vi "SUB-Calculation_Scale_of_CDC_by_data.vi"(10 "MAX r":dbl format="%#.6g", 11 "MIN r":dbl format="%#.6g") -> (3 "Scale(CDC)":dbl format="%#.6g")   [LabVIEW 2015]
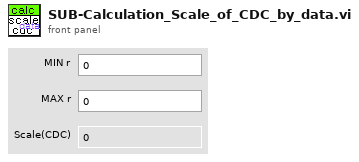
[diagram p1: front panel]
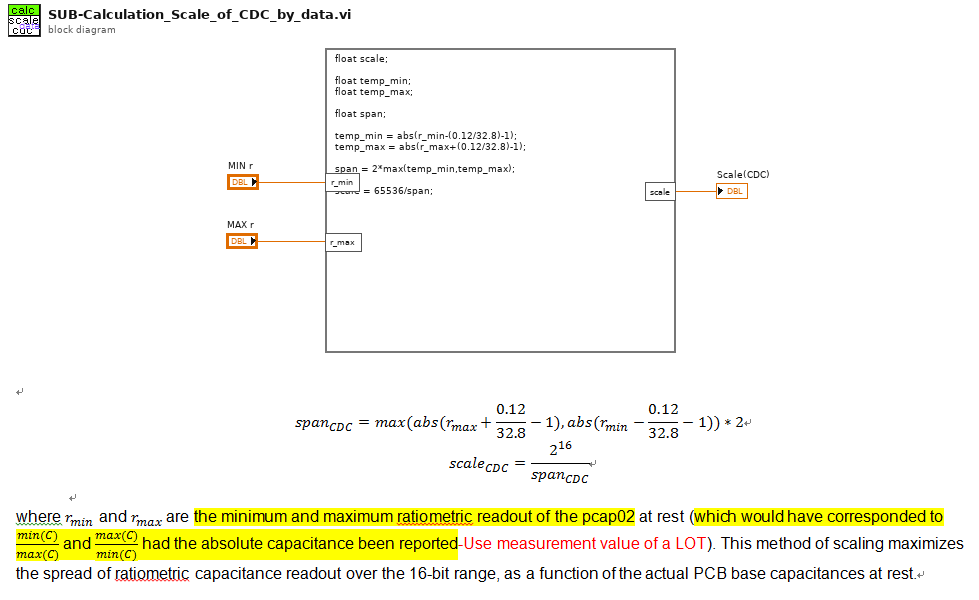
[diagram p0: block diagram]
diagram:
  n1 = formula code="float scale;\n\nfloat temp_min;\nfloat temp_max;\n\nfloat span;\n\ntemp_min = abs(r_min-(0.12/32.8)-1);\ntemp_max = abs(r_max+(0.12/32.8)-1);\n\nspan = 2*max(temp_min,temp_max);\n\nscale = 65536/span;"("r_min"="MIN r", "r_max"="MAX r") -> ("scale"=→"Scale(CDC)":dbl)
